vi "Manual_TDMScompress.vi"() -> ()   [LabVIEW 2012]
doc: "Writes a simulated signal to TDMS (Technical Data Management Streaming) file. Run this VI, then run the Read TDMS example to view the data."
uses:
  <vilib>/Utility/file.llb/Read From Spreadsheet File (DBL).vi
  <vilib>/Utility/file.llb/Read From Spreadsheet File (string).vi
panel:
  out "txt string":string
  in  "Path":path
  out "Channel Names":string[](array[string])
  # "This function writes a .txt file to a TDMS file. \n\nInstructions:\n1. Select the folder containing the .txt files you whish to convert\n2. Run this VI\n3. Select the TDMS File you wish to replace\n4. Use the Read TDMS example to view the data or look at the TDMS Viewer to see your data"
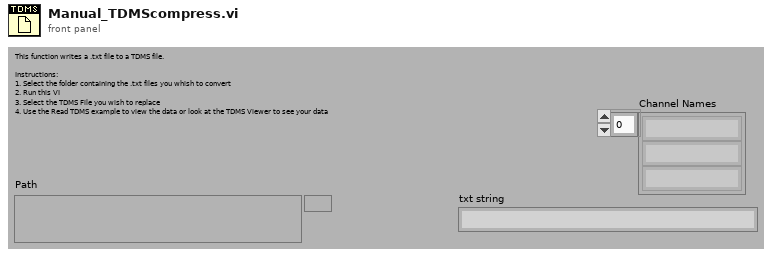
[diagram p1: front panel]
types:
  T1 = enum16{"open", "open or create", "create or replace", "create", "open (read-only)"}
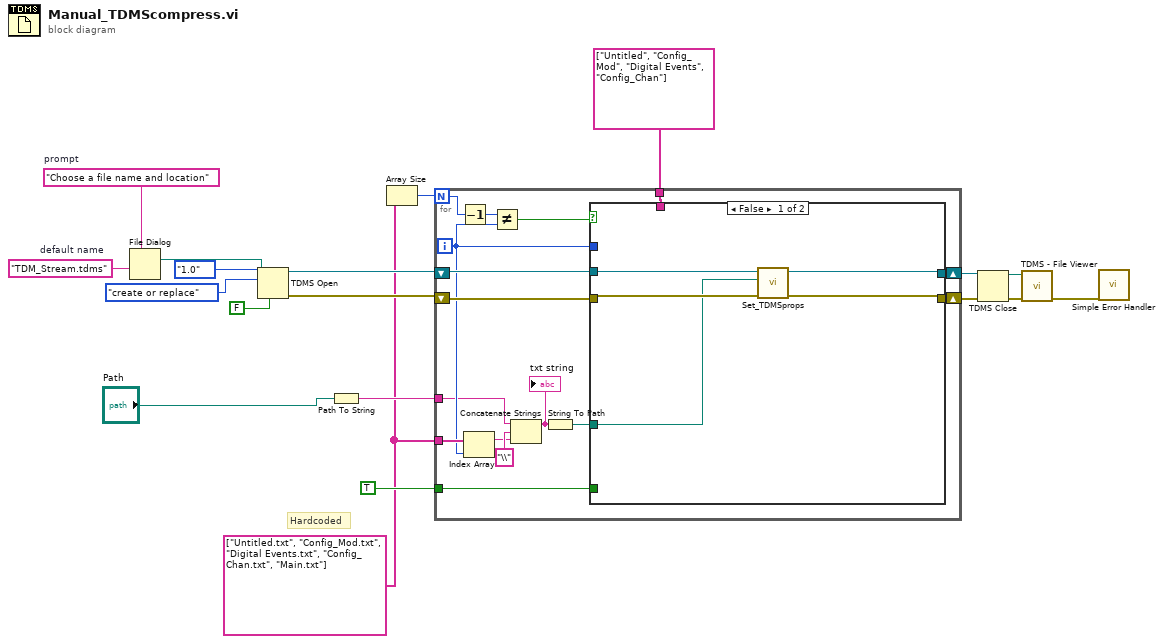
[diagram p0: block diagram]
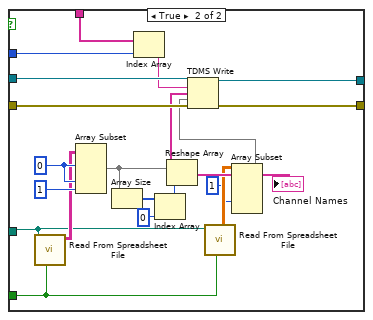
[diagram p2: hidden frame]
diagram:
  w1 = string[] ["Untitled.txt", "Config_Mod.txt", "Digital Events.txt", "Config_Chan.txt", "Main.txt"]
  w18 = "TDM_Stream.tdms"  # default name
  w19 = "Choose a file name and location"  # prompt
  # "Hardcoded"
  n1 = File Dialog(7:w19, 9:w18) -> (3:w17:path)  [unwired: 1 in, 7 out]
  n2 = TDMS Open(6:FALSE ("disable buffering (T)"), 7:enum16{"1.0", "2.0"}."1.0" ("file format version (2.0)"), 10:T1."create or replace" ("operation"), 11:w17) -> (0:w5:errorcluster, 3:w6:refnum<k34>)  [unwired: 2 in]
  n3 = Path To String(path="Path") -> (string=w10:string)
  n4 = Array Size(array=w1) -> (size(s)=w2:i32)
  n5 = for {
    N: w2 -> [w28]
    tunnel: TRUE ("transpose (no:F)") -> [w35]
    tunnel: string[] ["Untitled", "Config_Mod", "Digital Events", "Config_Chan"] -> [w34]
    tunnel: w10 -> [w22]
    shift-right: [w33] -> w9
    shift-left: w6 -> [w31]
    shift-right: [w32] -> w8
    shift-left: w5 -> [w30]
    tunnel: w1 -> [w25]
    i -> [w24]
    n6 = Decrement(x=w28) -> (x-1=w20:i32)
    n7 = Index Array(array=w25, index=w24) -> (element=w23:string)
    n8 = Not Equal?(x=w20, y=w24) -> (x != y?=w29:bool)
    n9 = Concatenate Strings(w22, "\\" ("string"), w23) -> (w27:string)
    "txt string" <- w27
    n10 = String To Path(string=w27) -> (path=w21:path)
    n11 = case shown="False" w29 {
      tunnel: w35 -> [_ w60]
      tunnel: w34 -> [_ w59]
      tunnel: [w39 w58] -> w33
      tunnel: [w38 w57] -> w32
      tunnel: w31 -> [w40 w56]
      tunnel: w30 -> [w37 w55]
      tunnel: w24 -> [_ w42]
      tunnel: w21 -> [w36 w41]
      frame False {
        n12 = call "Set_TDMSprops.vi"("error in (no error)"=w37, "Path"=w36, "tdms file"=w40) -> ("error out"=w38:errorcluster, "tdms file out"=w39:refnum<k34>)  [unwired: 7 in]
      }
      frame True {
        w54 = 0 ("index")
        n13 = call-poly <vilib>:"Read From Spreadsheet File.vi"("transpose (no:F)"=w60, "file path (dialog if empty)"=w41) -> ("all rows"=w52:string[][])  [unwired: 5 in, 4 out]
        n14 = Array Subset(array=w52, index (row)=w54, index (col)=w54, length (col)=1 ("length")) -> (w51:string[][])  [unwired: 1 in]
        n15 = Array Size(array=w51) -> (size(s)=w50:i32[])
        n16 = Index Array(array=w59, index=w42) -> (element=w46:string)
        n17 = Index Array(array=w50, index=0) -> (element=w49:i32)
        n18 = Reshape Array(w51, w49) -> (w47:string[])
        "Channel Names" <- w47
        n19 = call-poly <vilib>:"Read From Spreadsheet File.vi"("transpose (no:F)"=w60, "file path (dialog if empty)"=w41) -> ("all rows"=w45:dbl[][])  [unwired: 5 in, 4 out]
        n20 = Array Subset(array=w45, index (col)=1 ("index")) -> (w44:dbl[][])  [unwired: 3 in]
        n21 = TDMS Write(0:w56, 5:w46, 7:w47, 9:w44, 11:w55) -> (4:w58:refnum<k34>, 15:w57:errorcluster)  [unwired: 1 in, 2 out]
      }
    }
  }
  n22 = TDMS Close(8:w8, 11:w9) -> (0:w14:errorcluster, 3:w15:path)
  n23 = call <vilib>:"TDMS - File Viewer.vi"("error in (no error)"=w14, "file path"=w15) -> ("error out"=w13:errorcluster)  [unwired: 4 in, 1 out]
  n24 = call <vilib>:"Simple Error Handler.vi"("error in (no error)"=w13) -> ()  [unwired: 1 in, 8 out]
